vi "sub_dt-check.vi"() -> (2 "dt s":dbl, 3 "dt ms":u32)   [LabVIEW 2019]
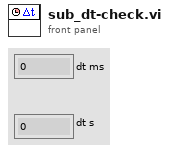
[diagram p1: front panel]
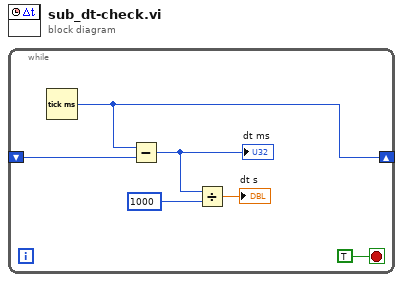
[diagram p0: block diagram]
diagram:
  n1 = while {
    shift-right: [w4] -> _
    shift-left: _ -> [w5]
    stop <- TRUE stop-if-true
    n2 = Tick Count (ms)() -> (millisecond timer value=w4:u32)
    n3 = Subtract(x=w4, y=w5) -> (x-y=w3:u32)
    "dt ms" <- w3
    n4 = Divide(x=w3, y=u32 1000) -> (x/y=→"dt s":dbl)
  }
